vi "Get Service Interface.vi"(8 "error in":errorcluster, 11 "measurement service in":refnum<class "IMeasurement Service.lvclass">) -> (0 "error out":errorcluster, 2 "service interface":string, 3 "measurement service out":refnum<class "IMeasurement Service.lvclass">)   [LabVIEW 2020, in "Measurement Plugin Measurement Server.lvlib" / "IMeasurement Service.lvclass"]
uses:
  IMeasurement Service.lvclass
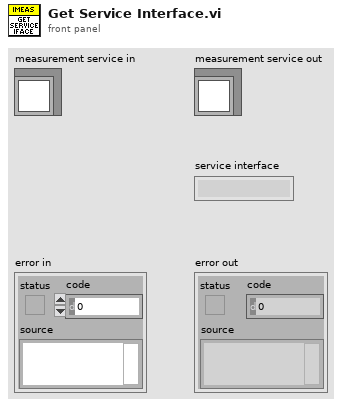
[diagram p1: front panel]
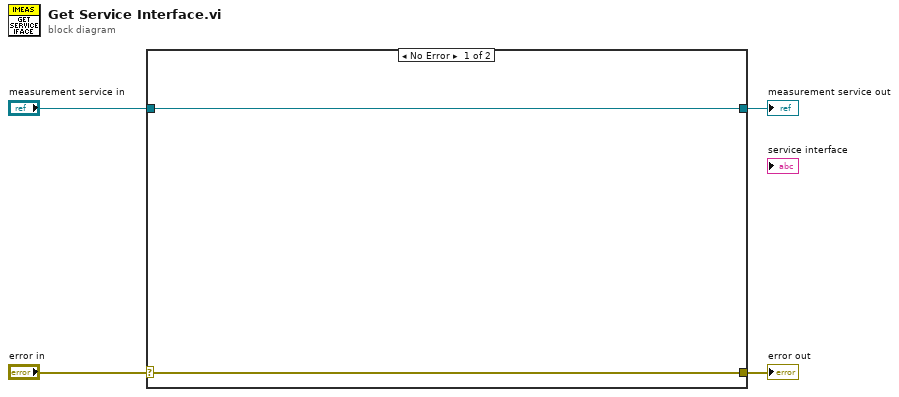
[diagram p0: block diagram]
diagram:
  n1 = case shown="No Error" "error in" {
    selector: "error in" -> [w5 w8]
    tunnel: [w5 w8] -> w3
    tunnel: [w6 w7] -> w1
    tunnel: "measurement service in" -> [w6 w7]
    frame No Error {
    }
    frame Error {
    }
  }
  "error out" <- w3
  "measurement service out" <- w1
